vi "TestExecuteOneShotSubscription_PublishOK.vi"(8 "error in (no error)":errorcluster, 11 "TestCase in":refnum<class "TestSubscriptionPolicy.lvclass">) -> (0 "error out":errorcluster, 3 "TestCase out":refnum<class "TestSubscriptionPolicy.lvclass">)   [LabVIEW 2015, in "SubscriptionPolicy.lvlib" / "TestSubscriptionPolicy.lvclass"]
uses:
  TestSubscriptionPolicy.lvclass
  OneShotSubscription/OneShotSubscription.lvclass/OneShotSubscription.ctl
  OneShotSubscription/OneShotSubscription.lvclass
  Transport/QueueTransport/QueueTransport.lvclass
  IMediator/ISubscriptionPolicy/ISubscriptionPolicy.lvclass
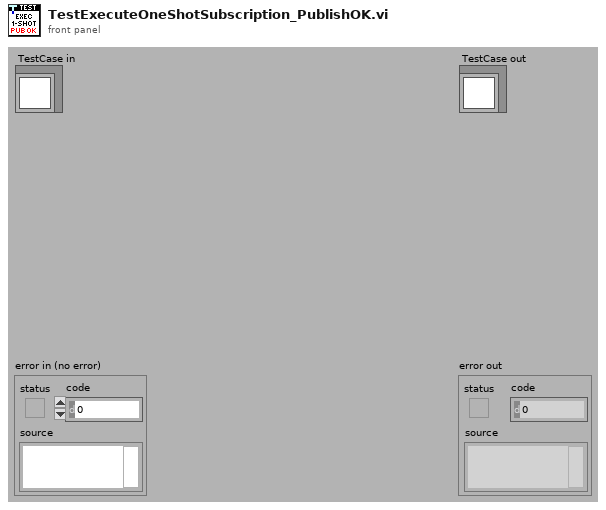
[diagram p1: front panel]
types:
  T1 = typedef "IMediator.lvlib/ISubscriptionPolicy.lvclass/ISubscriptionPolicy Reference.ctl" = refnum<data-value>
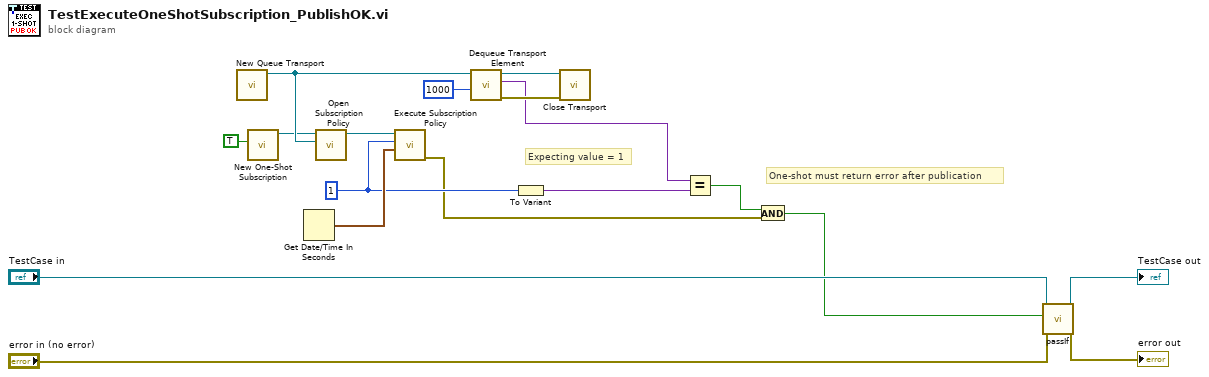
[diagram p0: block diagram]
diagram:
  w6 = 1
  # "One-shot must return error after publication"
  # "Expecting value = 1"
  n1 = call "New Queue Transport.vi"() -> ("QueueTransport Out"=w13:refnum<class "QueueTransport.lvclass">)  [unwired: 10 in, 1 out]
  n2 = call "New One-Shot Subscription.vi"("Ignore Past Updates? (F)"=TRUE) -> ("OneShotSubscription Out"=w8:refnum<class "OneShotSubscription.lvclass">)  [unwired: 10 in]
  n3 = Get Date/Time In Seconds() -> (seconds since 1Jan1904=w11:timestamp)
  n4 = call "Open Subscription Policy.vi"("Transport"=w13, "SubscriptionPolicy"=w8) -> ("Subscription Policy"=w14:T1)  [unwired: 8 in, 1 out]
  n5 = call "Execute Subscription Policy.vi"("Publish Time"=w11, "New Topic Value"=w6, "Subscription Policy"=w14) -> ("error out (Unsubscribe?)"=w3:errorcluster)  [unwired: 8 in]
  n6 = call "Dequeue Transport Element.vi"("Timeout In ms (-1)"=1000, "QueueTransport in"=w13) -> ("error out"=w9:errorcluster, "Data"=w1:variant, "QueueTransport out"=w10:refnum<class "QueueTransport.lvclass">)  [unwired: 6 in, 1 out]
  n7 = To Variant(anything=w6) -> (Variant=w5:variant)
  n8 = call-dynamic "Close Transport.vi"("error in (no error)"=w9, "QueueTransport in"=w10) -> ()  [unwired: 9 in, 1 out]
  n9 = Equal?(x=w1, y=w5) -> (x = y?=w4:bool)
  n10 = And(x=w4, y=w3) -> (x .and. y?=w2:bool)
  n11 = call-dynamic "passIf.vi"("error in (no error)"="error in (no error)", "pass"=w2, "TestCase in"="TestCase in") -> ("error out"=→"error out":errorcluster, "TestCase out"=→"TestCase out":refnum<class "TestSubscriptionPolicy.lvclass">)  [unwired: 7 in]
